vi "UI_Name.vi"(11 "Main VI":refnum<vi>) -> (2 "Vaild?":bool, 3 "Name Output":string)   [LabVIEW 2015, in "ConfigHelper.lvlib"]
uses:
  ConfigHelper.lvlib
panel:
  in  "Cancel":bool
  in  "OK":bool
  in  "String":string
  # "Name"
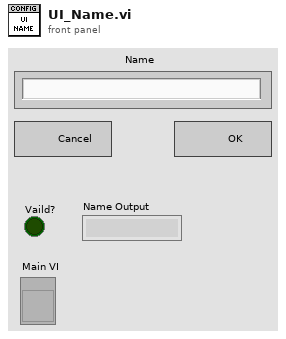
[diagram p1: front panel]
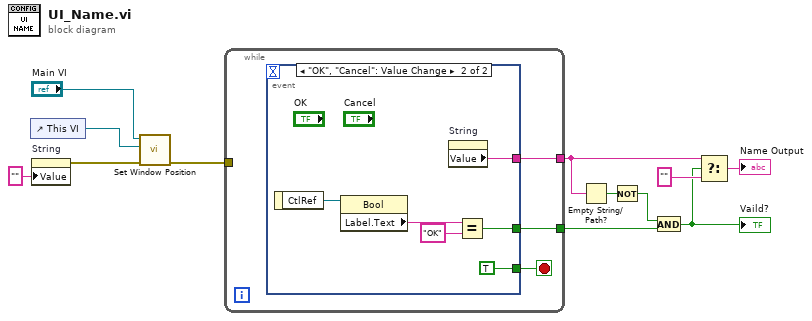
[diagram p0: block diagram]
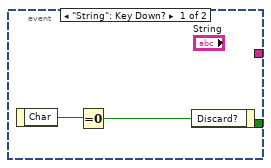
[diagram p2: hidden frame]
diagram:
  n1 = control-ref of="This VI"() -> (w1:refnum<vi>)
  n2 = property on="String" class="Str"("Value"="" ("String")) -> (error out=w4:errorcluster)  [unwired: 2 in, 1 out]
  n3 = call "Set Window Position.vi"("error in (no error)"=w4, "Current VI"=w1, "Main VI"="Main VI") -> ("error out"=w3:errorcluster)  [unwired: 8 in]
  n4 = while {
    tunnel: [w15] -> w10
    tunnel: [w13] -> w9
    tunnel: w3 -> [_]
    stop <- w14 stop-if-true
    n5 = event shown="[1] \"OK\", \"Cancel\": Value Change" {
      selector: _ -> [_ _]
      dyn-events: _ -> [_ _]
      timeout: _ -> [_ _]
      tunnel: [_ w20] -> w15
      tunnel: [_ TRUE] -> w14
      tunnel: [_ w18] -> w13
      event "String": Key Down? {
        n6 = event-data() -> ("Char"=w17:i16)  [unwired: 1 in]
        n7 = Equal To 0?(x=w17) -> (x = 0?=w16:bool)
        n8 = event-data("Discard?"=w16) -> ()  [unwired: 1 in, 1 out]
      }
      event "OK", "Cancel": Value Change {
        n9 = event-data() -> ("CtlRef"=w23:refnum<vi>)  [unwired: 1 in]
        n10 = property class="Bool"(reference=w23) -> ("Label.Text"=w22:string)  [unwired: 1 in, 2 out]
        n11 = property on="String" class="Str"() -> ("Value"=w18:string)  [unwired: 2 in, 2 out]
        n12 = Equal?(x=w22, y="OK") -> (x = y?=w20:bool)
      }
    }
  }
  n13 = Empty String/Path?(string/path=w9) -> (empty?=w11:bool)
  n14 = Not(x=w11) -> (.not. x?=w8:bool)
  n15 = And(x=w8, y=w10) -> (x .and. y?=w5:bool)
  "Vaild?" <- w5
  n16 = Select(t=w9, s=w5, f="") -> (s? t:f=→"Name Output":string)
